vi "Robot Global Data.vi"() -> ()   [LabVIEW 2016]
doc: "This global VI can contain as many global variables as you need. Place a control on the panel, give it a good name. To read or write to it from a VI, drag the icon to the diagram of that VI. You can also drag from the project. Click on the node to change which global you access. You shouldn't have multiple locations writing to a global or it will cause a race-condition."
uses:
  <vilib>/Rock Robotics/WPI/Camera/WPI_CameraImageSize.ctl
  <vilib>/Rock Robotics/WPI/DriverStation/WPI_DriverStationRobotMode2.ctl
panel:
  out "RPM Auto Trim":dbl=-4.190677999999786
  in  "Real Turret?":bool
  out "Good to Shoot?":bool=TRUE
  out "Slow Loop":u32=100
  out "Fast Loop":u32=40
  out "SensorPos (rotations)":dbl=-0.04773462783171521
  in  "Practice Robot?":bool
  out "Target X-value (norm)":dbl
  out "Gear Flap":bool
  out "Flashlight":bool
  out "Elevator-Down":bool=TRUE
  out "Process Vision":bool
  out "Vision Results":T1={"Distance (ft)"=nan, "Score"=0.0, "Normalized"={"Center"={nan, nan}, "Rectangle"={"Numeric"=nan, "Numeric 2"=nan, "Numeric 3"=nan, "Numeric 5"=nan}}, "Pixels"={"Center"={0.0, 0.0}, "Rectangle"={"Numeric"=0.0, "Numeric 2"=0.0, "Numeric 3"=0.0, "Numeric 5"=0.0}}} {"Score" format="%#_3g"; "Pixels"."Rectangle"."Numeric 5" format="%#_3g"; "Pixels"."Rectangle"."Numeric 3" format="%#_3g"; "Pixels"."Rectangle"."Numeric 2" format="%#_3g"; "Pixels"."Rectangle"."Numeric" format="%#_3g"; "Normalized"."Rectangle"."Numeric 5" format="%#_2g"; "Normalized"."Rectangle"."Numeric 3" format="%#_2g"; "Normalized"."Rectangle"."Numeric 2" format="%#_2g"; "Normalized"."Rectangle"."Numeric" format="%#_2g"; "Normalized"."Center"."?" format="%#_3g"; "Normalized"."Center"."?" format="%#_3g"; "Distance (ft)" format="%#_3g"}
  out "Turret Zero":bool
  out "Shooter Boost":dbl=-0.0
  out "Turret Course":dbl=-0.047244094488188976
  out "Launcher":dbl=1.0
  out "Yaw":dbl=-4.190677999999786
  out "Navx reading":bool
  out "Flywheel RPM":dbl=3000.0
  out "Target X-value (dg)":dbl=-0.12598425196850394
  out "Vision":bool
  out "Shoot-Back":bool
  out "IntakeIn":dbl
  out "Launcher Auto":bool
  out "Turret Auto":bool
  out "Elevator":bool
  out "Intake-Out":bool
  out "Climber-Up":bool
  out "Shoot":bool
  out "Intake-In":bool
  out "Y-Axis":dbl=0.007874015748031496
  out "Z-Axis":dbl=-2.1700043400086797e-05
  in  "Robot Mode":T2=enum."Teleop Disabled"
  in  "image size":T3=enum."320x240"
  in  "Enable Vision":bool=TRUE
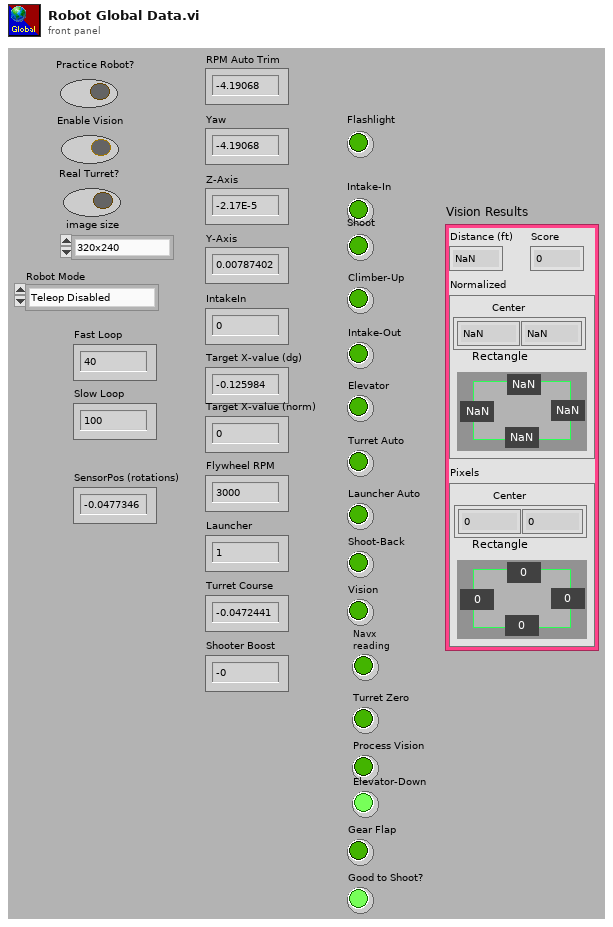
[diagram p1: front panel]
types:
  T1 = cluster{"Distance (ft)":dbl, "Score":dbl, "Normalized":cluster{"Center":cluster{dbl, dbl}, "Rectangle":cluster{"Numeric":dbl, "Numeric 2":dbl, "Numeric 3":dbl, "Numeric 5":dbl}}, "Pixels":cluster{"Center":cluster{dbl, dbl}, "Rectangle":cluster{"Numeric":dbl, "Numeric 2":dbl, "Numeric 3":dbl, "Numeric 5":dbl}}}
  T2 = typedef "WPI_DriverStationRobotMode2.ctl" = enum16{"Autonomous Disabled", "Autonomous Enabled", "Teleop Disabled", "Teleop Enabled", "Disconnected", "Finish", "Test Disabled", "Test Enabled", "Emergency Stopped"}
  T3 = typedef "WPI_CameraImageSize.ctl" = enum16{"640x480", "320x240", "160x120", "Custom"}
diagram:
